vi "4155C START single.vi"(4 "error in (no error)":errorcluster, 5 "Emergency Stop":refnum<vi>, 7 "VISA resource name in":refnum<visa-resource-name>) -> (0 "error out":errorcluster, 3 "VISA Resource Name out":refnum<visa-resource-name>)   [LabVIEW 2016]
uses:
  Select Event Type.ctl
panel:
  in  "event resource class":refnum<visa-resource-name>
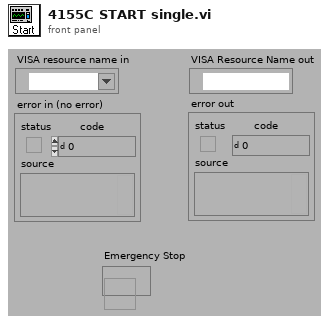
[diagram p1: front panel]
types:
  T1 = typedef "Select Event Type.ctl" = u32
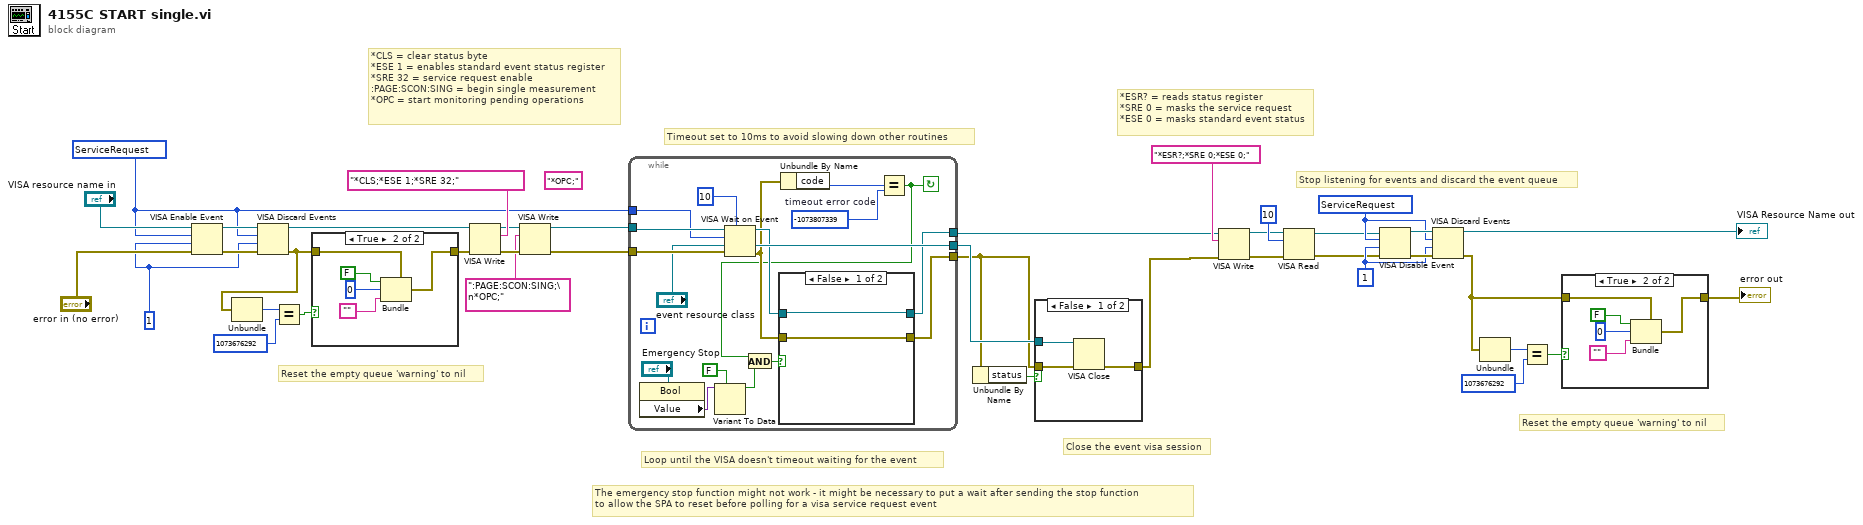
[diagram p0: block diagram]
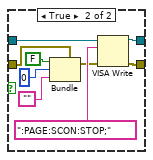
[diagram p2: hidden frame]
diagram:
  (unwired) "*OPC;" ("write buffer (\"\")")
  w23 = u16 1
  w24 = T1 1073684491 items=["ServiceRequest"=1073684491, "Trigger"=3221168138, "Clear"=1073684493, "VXI-Signal"=1073684512, "VXI/VME-Interrupt"=3221168161, "VXI/VME-Sysfail"=1073684509, "VXI/VME-Sysreset"=1073684510, "GPIB-CIC"=1073684498, "GPIB-Talk"=1073684499, "GPIB-Listen"=1073684500, "PXI-Interrupt"=1073684514, "AllEnabled"=1073709055]
  w32 = T1 1073684491 items=["ServiceRequest"=1073684491, "Trigger"=3221168138, "Clear"=1073684493, "VXI-Signal"=1073684512, "VXI/VME-Interrupt"=3221168161, "VXI/VME-Sysfail"=1073684509, "VXI/VME-Sysreset"=1073684510, "GPIB-CIC"=1073684498, "GPIB-Talk"=1073684499, "GPIB-Listen"=1073684500, "PXI-Interrupt"=1073684514, "AllEnabled"=1073709055] ("Event Type")
  w36 = u32 1 ("mechanism (1:  VI_QUEUE)")
  # "Reset the empty queue 'warning' to nil"
  # "Stop listening for events and discard the event queue"
  # "The emergency stop function might not work - it might be necessary to put a wait after sending the stop function\nto allow the SPA to reset before polling for a visa service request event"
  # "*ESR? = reads status register\n*SRE 0 = masks the service request\n*ESE 0 = masks standard event status"
  # "Reset the empty queue 'warning' to nil"
  # "Timeout set to 10ms to avoid slowing down other routines"
  # "Close the event visa session"
  # "Loop until the VISA doesn't timeout waiting for the event"
  # "*CLS = clear status byte\n*ESE 1 = enables standard event status register\n*SRE 32 = service request enable\n:PAGE:SCON:SING = begin single measurement\n*OPC = start monitoring pending operations"
  n1 = VISA Enable Event(8:"error in (no error)", 9:w36, 10:w32, 11:"VISA resource name in") -> (0:w37:errorcluster, 3:w35:refnum<visa-resource-name>)
  n2 = VISA Discard Events(8:w37, 9:w36, 10:w32, 11:w35) -> (0:w6:errorcluster, 3:w34:refnum<visa-resource-name>)
  n3 = Unbundle(w6) -> ("code"=w9:i32)  [unwired: 2 out]
  n4 = Equal?(x=w9, y=1073676292) -> (x = y?=w7:bool)
  n5 = case shown="True" w7 {
    tunnel: w6 -> [w40 w45]
    tunnel: [w40 w44] -> w5
    frame False {
    }
    frame True {
      n6 = Bundle(cluster=w45, "status"=FALSE, "code"=0, "source"="") -> (w44:errorcluster)
    }
  }
  n7 = VISA Write(VISA resource name=w34, write buffer="*CLS;*ESE 1;*SRE 32;" ("write buffer (\"\")"), error in (no error)=w5) -> (VISA resource name out=w13:refnum<visa-resource-name>, error out=w14:errorcluster)  [unwired: 1 out]
  n8 = VISA Write(VISA resource name=w13, write buffer=":PAGE:SCON:SING;\n*OPC;" ("write buffer (\"\")"), error in (no error)=w14) -> (VISA resource name out=w4:refnum<visa-resource-name>, error out=w3:errorcluster)  [unwired: 1 out]
  n9 = while {
    tunnel: [w54] -> w1
    tunnel: [w55] -> w10
    tunnel: [w58] -> w15
    tunnel: w32 -> [w60]
    tunnel: w3 -> [w62]
    tunnel: w4 -> [w63]
    stop <- w50 continue-if-true
    w56 = -1073807339  # timeout error code
    n10 = property class="Bool"(reference="Emergency Stop") -> ("Value"=w48:variant)  [unwired: 1 in, 2 out]
    n11 = Variant To Data(type=FALSE, Variant=w48) -> (data=w47:bool)  [unwired: 1 in, 1 out]
    n12 = VISA Wait on Event(7:u32 10 ("timeout (0)"), 8:w62, 9:"event resource class", 10:w60, 11:w63) -> (0:w52:errorcluster, 1:w58:refnum<visa-resource-name>, 3:w53:refnum<visa-resource-name>)  [unwired: 1 out]
    n13 = Unbundle By Name(w52) -> ("code"=w57:i32)
    n14 = Equal?(x=w57, y=w56) -> (x = y?=w50:bool)
    n15 = And(x=w50, y=w47) -> (x .and. y?=w51:bool)
    n16 = case shown="False" w51 {
      tunnel: w52 -> [w64 w70]
      tunnel: w53 -> [w65 w72]
      tunnel: [w65 w73] -> w54
      tunnel: [w64 w74] -> w55
      frame False {
      }
      frame True {
        n17 = Bundle(cluster=w70, "status"=FALSE, "code"=0, "source"="") -> (w66:errorcluster)
        n18 = VISA Write(VISA resource name=w72, write buffer=":PAGE:SCON:STOP;" ("write buffer (\"\")"), error in (no error)=w66) -> (VISA resource name out=w73:refnum<visa-resource-name>, error out=w74:errorcluster)  [unwired: 1 out]
      }
    }
  }
  n19 = Unbundle By Name(w10) -> ("status"=w31:bool)
  n20 = case shown="False" w31 {
    tunnel: w15 -> [w77 _]
    tunnel: w10 -> [w76 w78]
    tunnel: [w75 w78] -> w2
    frame False {
      n21 = VISA Close(VISA resource name=w77, error in (no error)=w76) -> (error out=w75:errorcluster)
    }
    frame True {
    }
  }
  n22 = VISA Write(VISA resource name=w1, write buffer="*ESR?;*SRE 0;*ESE 0;" ("write buffer (\"\")"), error in (no error)=w2) -> (VISA resource name out=w28:refnum<visa-resource-name>, error out=w27:errorcluster)  [unwired: 1 out]
  n23 = VISA Read(VISA resource name=w28, byte count=u32 10, error in (no error)=w27) -> (VISA resource name out=w18:refnum<visa-resource-name>, error out=w17:errorcluster)  [unwired: 2 out]
  n24 = VISA Disable Event(8:w17, 9:w23, 10:w24, 11:w18) -> (0:w25:errorcluster, 3:w26:refnum<visa-resource-name>)
  n25 = VISA Discard Events(8:w25, 9:w23, 10:w24, 11:w26) -> (0:w19:errorcluster, 3:→"VISA Resource Name out":refnum<visa-resource-name>)
  n26 = Unbundle(w19) -> ("code"=w22:i32)  [unwired: 2 out]
  n27 = Equal?(x=w22, y=1073676292) -> (x = y?=w20:bool)
  n28 = case shown="True" w20 {
    tunnel: w19 -> [w79 w84]
    tunnel: [w79 w83] -> w11
    frame False {
    }
    frame True {
      n29 = Bundle(cluster=w84, "status"=FALSE, "code"=0, "source"="") -> (w83:errorcluster)
    }
  }
  "error out" <- w11
